vi "Register Self.vi"(8 "error in (no error)":errorcluster, 11 "CO2 Actor in":refnum<class "CO2 Actor.lvclass">) -> (0 "error out":errorcluster, 3 "CO2 Actor out":refnum<class "CO2 Actor.lvclass">)   [LabVIEW 2015, in "cRIO-Carbondioxide.lvlib" / "CO2-Actor.lvlib" / "CO2 Actor.lvclass"]
uses:
  CO2 Actor.lvclass
  cRIO-CO2 Messages/Register Actor Msg/Register Actor Msg.lvclass/Register Actor Msg.ctl
  <vilib>/ActorFramework/Message Enqueuer/Message Enqueuer.lvclass/Message Enqueuer.ctl
  <vilib>/ActorFramework/Message Enqueuer/Enqueue.vi
  <vilib>/ActorFramework/Message Priority Queue/Priority Enqueue.vi
  cRIO-CO2 Messages/Register Actor Msg/Register Actor Msg.lvclass
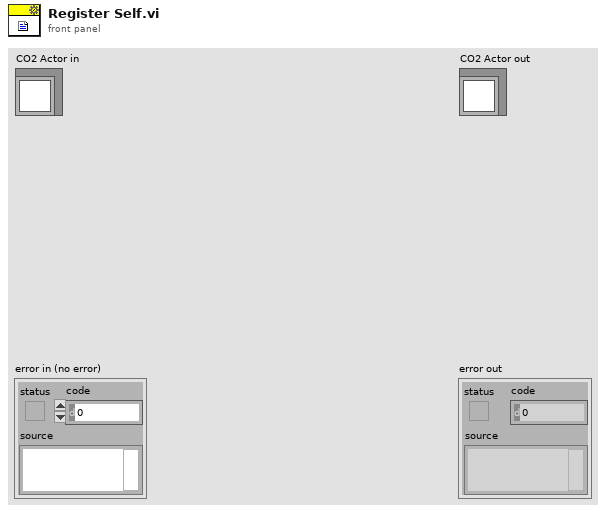
[diagram p1: front panel]
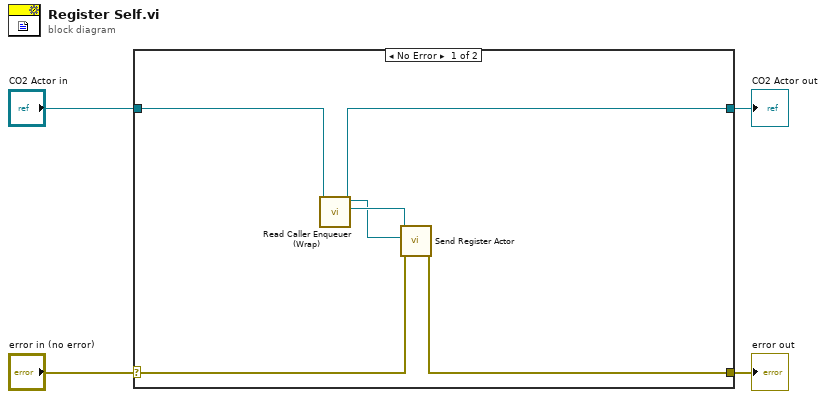
[diagram p0: block diagram]
diagram:
  n1 = case shown="No Error" "error in (no error)" {
    selector: "error in (no error)" -> [w6 w11]
    tunnel: [w5 w11] -> w3
    tunnel: [w7 w10] -> w1
    tunnel: "CO2 Actor in" -> [w8 w10]
    frame No Error {
      n2 = call "Read Caller Enqueuer (Wrap).vi"("CO2 Actor in"=w8) -> ("Actor Framework:Message Enqueuer"=w9:refnum<class "Message Enqueuer.lvclass">, "CO2 Actor out"=w7:refnum<class "CO2 Actor.lvclass">)  [unwired: 9 in]
      n3 = call "Send Register Actor.vi"("error in (no error)"=w6, "CO2 Actor"=w7, "Message Enqueuer"=w9) -> ("error out"=w5:errorcluster)  [unwired: 7 in, 1 out]
    }
    frame Error {
    }
  }
  "error out" <- w3
  "CO2 Actor out" <- w1
